vi "Keithley 2450 Source V read I.vi"() -> ()   [LabVIEW 2024]
doc: "This example shows how to configure a measurement and take multiple readings."
uses:
  C:/Users/Public/OneDrive/Desktop/Keithley_2450_2470_1_4_0_LV2015_NewReadme2_2450-LV2015-1.4.0/Keithley 2450/Keithley 2450.lvlib
panel:
  in  "Compliance Level (0.1)":dbl=0.1
  in  "Output Level (0)":dbl
  in  "Source Mode  (0: Voltage)":u16(ring) items=["Voltage", "Current"]
  out "Current":sgl[](array[numeric])
  in  "VISA resource name":refnum<visa-resource-name>
  # "(c) 2021 National Instruments.  ALL RIGHTS RESERVED."
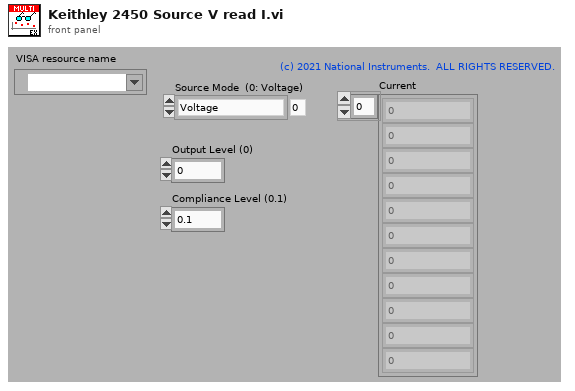
[diagram p1: front panel]
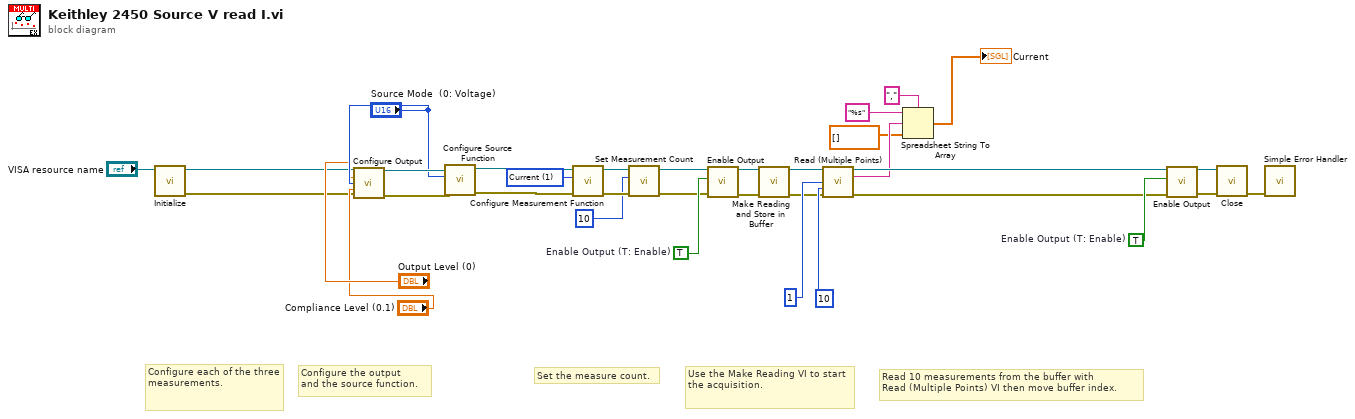
[diagram p0: block diagram]
diagram:
  w1 = u16 1 items=["Volts", "Current", "Auto Resistance", "Manual Resistance", "Digitize Voltage", "Digitize Current"] ("Function (0: Volts)")
  w6 = TRUE  # Enable Output (T: Enable)
  w30 = TRUE  # Enable Output (T: Enable)
  # "Read 10 measurements from the buffer with \nRead (Multiple Points) VI then move buffer index."
  # "Set the measure count."
  # "Use the Make Reading VI to start the acquisition."
  # "Configure the output \nand the source function."
  # "Configure each of the three measurements."
  n1 = call "Initialize.vi"("VISA resource name"="VISA resource name") -> ("error out"=w19:errorcluster, "VISA resource name out"=w20:refnum<visa-resource-name>)  [unwired: 9 in]
  n2 = call "Configure Output.vi"("VISA resource name"=w20, "Source Level (0)"="Output Level (0)", "Source Mode  (0: Voltage)"="Source Mode  (0: Voltage)", "Source Limit Level (0.1)"="Compliance Level (0.1)", "error in (no error)"=w19) -> ("VISA resource name out"=w26:refnum<visa-resource-name>, "error out"=w27:errorcluster)  [unwired: 9 in]
  n3 = call "Configure Source Function.vi"("error in (no error)"=w27, "Function (0: Volts)"="Source Mode  (0: Voltage)", "VISA resource name"=w26) -> ("error out"=w24:errorcluster, "VISA resource name out"=w25:refnum<visa-resource-name>)  [unwired: 7 in]
  n4 = call "Configure Measurement Function.vi"("error in (no error)"=w24, "Function (0: Volts)"=w1, "VISA resource name"=w25) -> ("error out"=w18:errorcluster, "VISA resource name out"=w17:refnum<visa-resource-name>)  [unwired: 7 in]
  n5 = call "Set Measurement Count.vi"("error in (no error)"=w18, "Measurement Count"=u32 10 ("millisecond multiple"), "VISA resource name"=w17) -> ("error out"=w4:errorcluster, "VISA resource name out"=w5:refnum<visa-resource-name>)  [unwired: 7 in]
  n6 = call "Enable Output.vi"("error in (no error)"=w4, "Enable Output (T: Enable)"=w6, "VISA resource name"=w5) -> ("error out"=w2:errorcluster, "VISA resource name out"=w3:refnum<visa-resource-name>)  [unwired: 7 in]
  n7 = call "Make Reading and Store in Buffer.vi"("VISA resource name"=w3, "error in (no error)"=w2) -> ("VISA resource name out"=w8:refnum<visa-resource-name>, "error out"=w7:errorcluster)  [unwired: 12 in]
  n8 = call "Read (Multiple Points).vi"("VISA resource name"=w8, "Start Index (1)"=u32 1 ("millisecond multiple"), "End Index (1)"=u32 10 ("millisecond multiple"), "error in (no error)"=w7) -> ("VISA resource name out"=w29:refnum<visa-resource-name>, "Data out"=w15:string, "error out"=w28:errorcluster)  [unwired: 9 in]
  n9 = Spreadsheet String To Array(delimiter (Tab)=",", format string="%s", spreadsheet string=w15, array type (2D Dbl)=dbl[] []) -> (array=→"Current":dbl[])
  n10 = call "Enable Output.vi"("error in (no error)"=w28, "Enable Output (T: Enable)"=w30, "VISA resource name"=w29) -> ("error out"=w31:errorcluster, "VISA resource name out"=w32:refnum<visa-resource-name>)  [unwired: 7 in]
  n11 = call "Close.vi"("error in (no error)"=w31, "VISA resource name"=w32) -> ("error out"=w34:errorcluster)  [unwired: 9 in]
  n12 = call <vilib>:"Simple Error Handler.vi"("error in (no error)"=w34) -> ()  [unwired: 4 in, 5 out]
